vi "FB_MFA_StepperMove -NxtMv Axis1.vi"(11 "Position Put":sgl) -> (2 "DoGOError":bool, 3 "SetMoveError":bool)   [LabVIEW 2011]
panel:
  out "AAABuild 2":i32
  out "nAxis1":i16
  out "error AAABuild":errorcluster
  out "error SetUSBlink":errorcluster
  out "AAABuild":i32
  in  "error in":errorcluster
  in  "MintController":refnum<k7>(container)
  out "error Position Get":errorcluster
  out "error Position Put":errorcluster
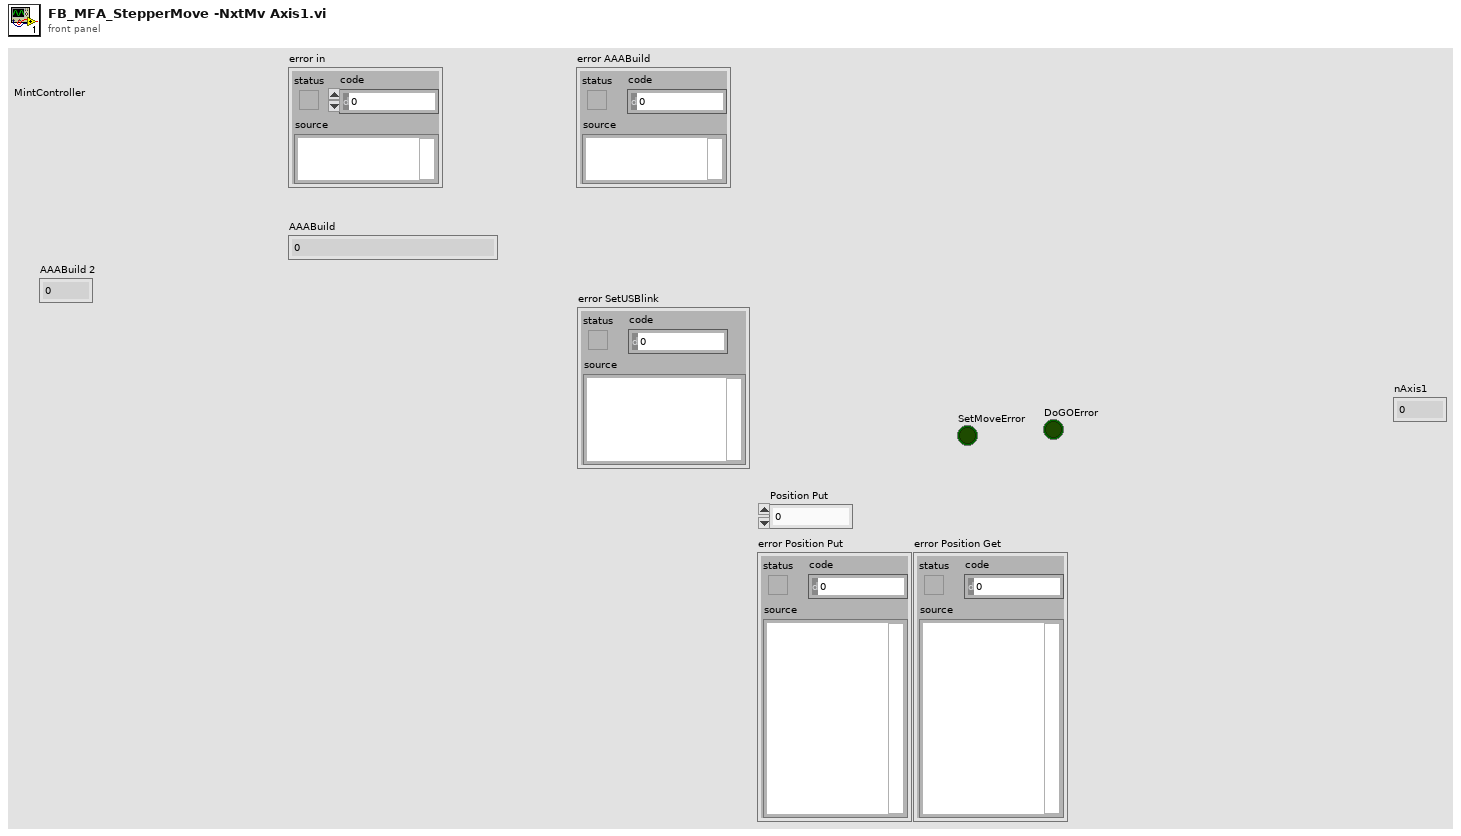
[diagram p1: front panel]
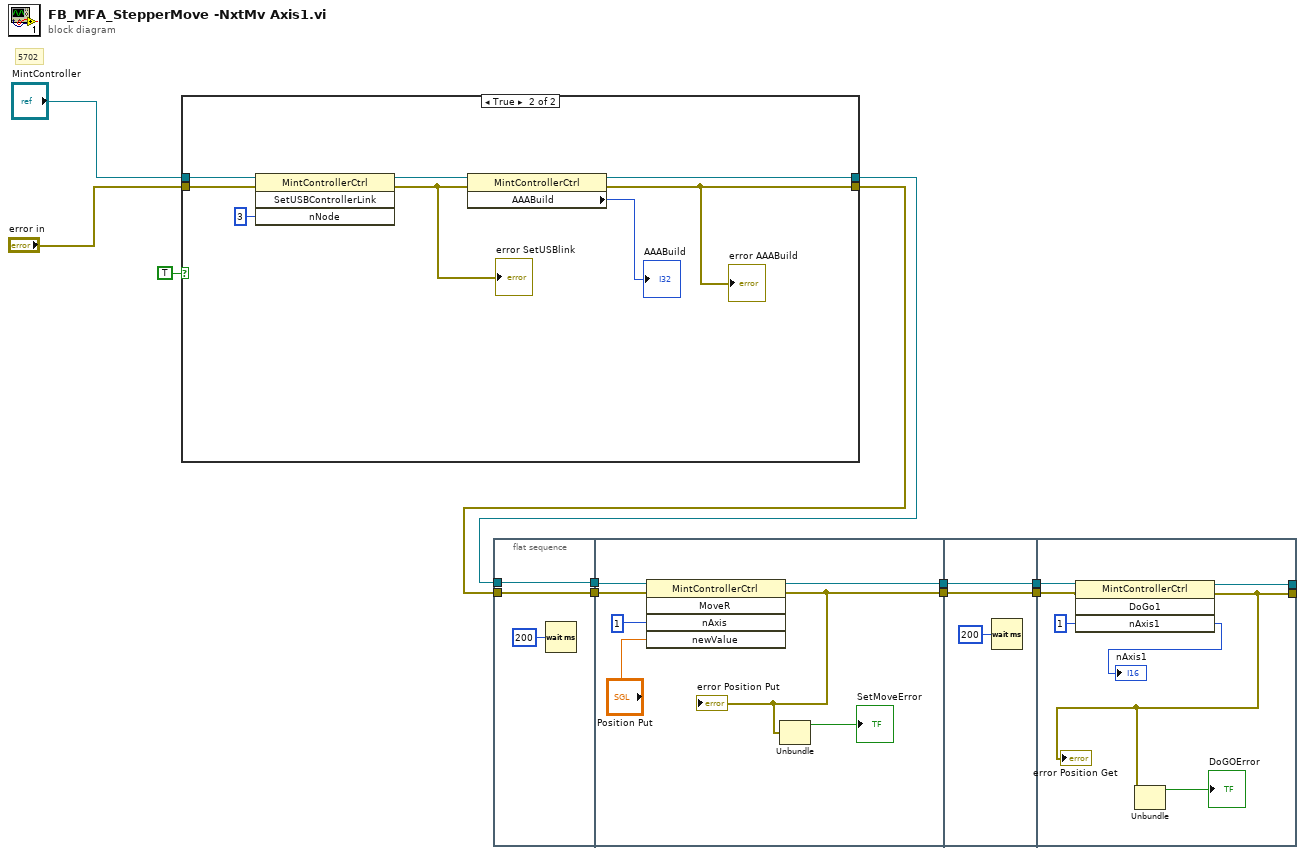
[diagram p0: block diagram]
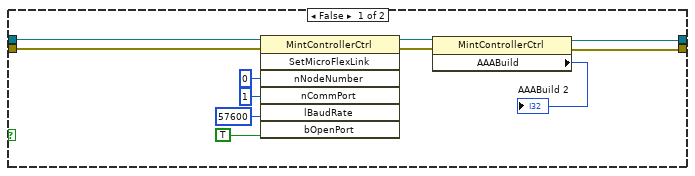
[diagram p2: hidden frame]
diagram:
  # "5702"
  n1 = case shown="True" TRUE {
    tunnel: "MintController" -> [w15 w30]
    tunnel: "error in" -> [w14 w29]
    tunnel: [w13 w24] -> w3
    tunnel: [w12 w23] -> w2
    frame False {
      n2 = invoke class="MintControllerCtrl" method="SetMicroFlexLink"(reference=w15, error in=w14, "nNodeNumber"=i16 0, "nCommPort"=i16 1, "lBaudRate"=57600, "bOpenPort"=TRUE) -> (reference out=w22:refnum<k7>, error out=w17:errorcluster)  [unwired: 1 in, 5 out]
      n3 = property class="MintControllerCtrl"(reference=w22, error in=w17) -> (reference out=w13:refnum<k7>, error out=w12:errorcluster, "AAABuild"=→"AAABuild 2":i32)
    }
    frame True {
      n4 = invoke class="MintControllerCtrl" method="SetUSBControllerLink"(reference=w30, error in=w29, "nNode"=i16 3) -> (reference out=w26:refnum<k7>, error out=w25:errorcluster)  [unwired: 1 in, 2 out]
      "error SetUSBlink" <- w25
      n5 = property class="MintControllerCtrl"(reference=w26, error in=w25) -> (reference out=w24:refnum<k7>, error out=w23:errorcluster, "AAABuild"=→"AAABuild":i32)
      "error AAABuild" <- w23
    }
  }
  n6 = flat-sequence {
    tunnel: [w33] -> w11
    tunnel: [w32] -> w10
    tunnel: w2 -> [w33]
    tunnel: w3 -> [w32]
    tunnel: w11 -> [w39]
    tunnel: w10 -> [w38]
    tunnel: [w37] -> w9
    tunnel: [w35] -> w8
    tunnel: w9 -> [w43]
    tunnel: w8 -> [w42]
    tunnel: [w43] -> w7
    tunnel: [w42] -> w6
    tunnel: w7 -> [w50]
    tunnel: w6 -> [w49]
    tunnel: [w47] -> _
    tunnel: [w44] -> _
    frame #0 {
      n7 = Wait (ms)(milliseconds to wait=u32 200) -> ()  [unwired: 1 out]
    }
    frame #1 {
      n8 = invoke class="MintControllerCtrl" method="MoveR"(reference=w38, error in=w39, "nAxis"=i16 1, "newValue"="Position Put") -> (reference out=w37:refnum<k7>, error out=w35:errorcluster)  [unwired: 1 in, 3 out]
      "error Position Put" <- w35
      n9 = Unbundle(w35) -> ("status"=→"SetMoveError":bool)  [unwired: 2 out]
    }
    frame #2 {
      n10 = Wait (ms)(milliseconds to wait=u32 200) -> ()  [unwired: 1 out]
    }
    frame #3 {
      n11 = invoke class="MintControllerCtrl" method="DoGo1"(reference=w50, error in=w49, "nAxis1"=i16 1 ("nBank")) -> (reference out=w47:refnum<k7>, error out=w44:errorcluster, "nAxis1"=→"nAxis1":i16)  [unwired: 1 in, 1 out]
      "error Position Get" <- w44
      n12 = Unbundle(w44) -> ("status"=→"DoGOError":bool)  [unwired: 2 out]
    }
  }
